vi "Base64.FileToBase64.vi"(8 "error in":errorcluster, 11 "Path":path) -> (0 "error out":errorcluster, 3 "Base64String":string)   [LabVIEW 2019]
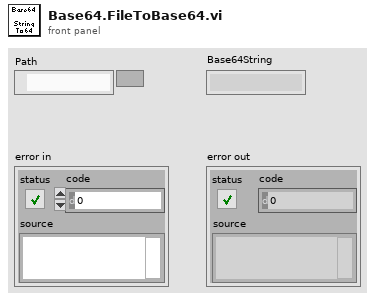
[diagram p1: front panel]
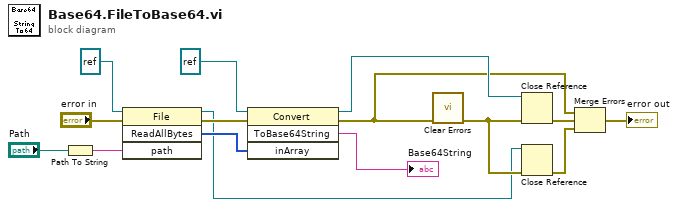
[diagram p0: block diagram]
diagram:
  n1 = Path To String(path="Path") -> (string=w12:string)
  n2 = invoke class="File" method="ReadAllBytes"(reference=refnum<k24> refnum, error in="error in", "path"=w12) -> (reference out=w1:refnum<k24>, error out=w10:errorcluster, "ReadAllBytes"=w8:u8[])  [unwired: 1 in, 1 out]
  n3 = invoke class="Convert" method="ToBase64String"(reference=refnum<k24> refnum, error in=w10, "inArray"=w8) -> (reference out=w5:refnum<k24>, error out=w4:errorcluster, "ToBase64String"=→"Base64String":string)  [unwired: 1 in, 1 out]
  n4 = call <vilib>:"Clear Errors.vi"("error in (no error)"=w4) -> ("error out"=w2:errorcluster)  [unwired: 5 in, 1 out]
  n5 = Close Reference(reference=w5, error in (no error)=w2) -> (error out=w7:errorcluster)
  n6 = Close Reference(reference=w1, error in (no error)=w2) -> (error out=w3:errorcluster)
  n7 = Merge Errors(w4, w7, w3) -> (→"error out":errorcluster)
